vi "kal-test-elev-system.vi"() -> (0 "Error":bool, 3 "ElevatorSystem":T1)   [LabVIEW 2019]
uses:
  <vilib>/Rock Robotics/WPI/ThirdParty/JAS_Junk/TrajLib/Trajectory_Library.lvlib
  <vilib>/Analysis/Matrix/Datatypes/RealMatrix.ctl
  <vilib>/Analysis/Matrix/NI_Matrix.lvlib
  <vilib>/Rock Robotics/WPI/ThirdParty/JAS_Junk/TrajLib/LINEAR_SYSTEM.ctl
panel:
  # "<States,States>"
  # "<States,Inputs>"
  # "<Outputs,States>"
  # "<Outputs,Inputs>"
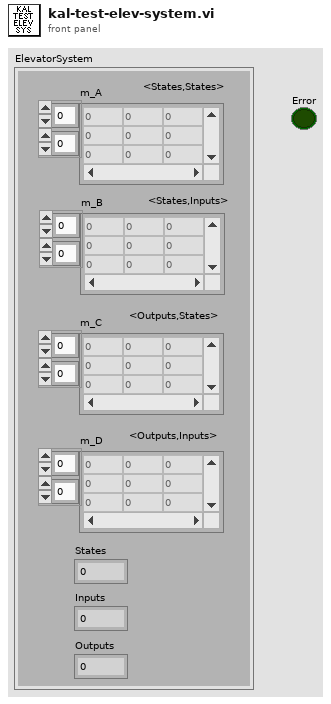
[diagram p1: front panel]
types:
  T1 = typedef "Trajectory_Library.lvlib/LINEAR_SYSTEM.ctl" = cluster{"m_A":T2, "m_B":T2, "m_C":T2, "m_D":T2, "States":i32, "Inputs":i32, "Outputs":i32}
  T2 = typedef "NI_Matrix.lvlib/RealMatrix.ctl" = dbl[][]
  T3 = typedef "Trajectory_Library.lvlib/DCMOTOR.CTL" = cluster{"nominalVoltage_Volts":dbl, "StallTorque_NM":dbl, "StallCurrent_Amps":dbl, "FreeCurrent_Amps":dbl, "FreeSpeed_RadPerSec":dbl, "R_Ohms":dbl, "Kv_RadPerSecPerVolt":dbl, "Kt_NMPerAmp":dbl}
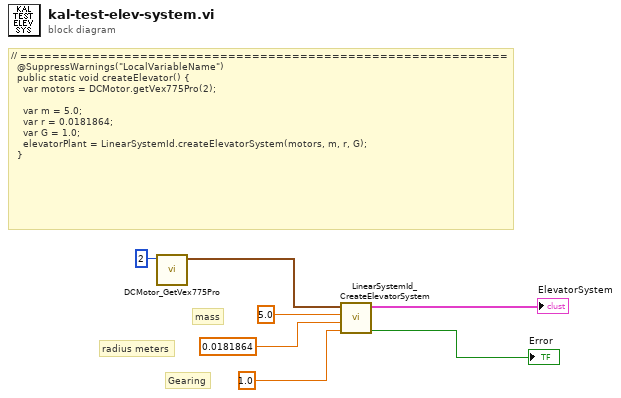
[diagram p0: block diagram]
diagram:
  # "Gearing"
  # "radius meters"
  # "mass"
  # "// =============================================================\n  @SuppressWarnings(\"LocalVariableName\")\n  public static void createElevator() {\n    var motors = DCMotor.getVex775Pro(2);\n\n    var m = 5.0;\n    var r = 0.0181864;\n    var G = 1.0;\n    elevatorPlant = LinearSystemId.createElevatorSystem(motors, m, r, G);\n  }"
  n1 = call <vilib>:"DCMotor_GetVex775Pro.vi"("Num Motors"=2) -> ("DCMOTOR"=w3:T3)  [unwired: 10 in]
  n2 = call <vilib>:"LinearSystemId_CreateElevatorSystem.vi"("G"=1.0, "radiusMeters"=0.0181864, "massKg"=5.0, "DCMOTOR"=w3) -> ("Size Coerced"=→"Error":bool, "Linearsystem"=→"ElevatorSystem":T1)  [unwired: 6 in]
